vi "AOL Z Cal load-Request to front.vi"(8 "error in (no error)":errorcluster) -> (0 "error out":errorcluster)   [LabVIEW 2020]
uses:
  Configuration code/Calibration/Globals/gl_Calibration globals.vi
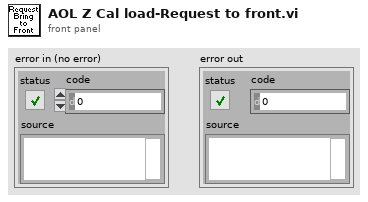
[diagram p1: front panel]
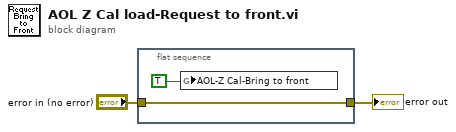
[diagram p0: block diagram]
diagram:
  n1 = flat-sequence {
    tunnel: "error in (no error)" -> [w4]
    tunnel: [w4] -> w2
    frame #0 {
      n2 = global write "gl_Calibration globals.vi" "AOL-Z Cal-Bring to front"(TRUE ("Bring to front")) -> ()
    }
  }
  "error out" <- w2
